vi "GEA3 Determine Valve Absolute Position.vi"(8 "error in (no error)":errorcluster, 9 "Target Position":i16, 11 ".NET Refnum in":refnum<k24>) -> (0 "error out":errorcluster, 1 "Valve Offset":i16, 3 ".NET Refnum out":refnum<k24>, 4 "Previous Mix Valve Position":u16)   [LabVIEW 2016]
uses:
  C:/TechnologyLab/NI-2010/Drivers/GEA3 Toolkit/GEA3 DLL Source/GeaCommunication.dll
  GEA3 DLL Source/GeaCommunication.dll
panel:
  out "Valve Offset Debug":i16
  in  "Current Position Debug":i16
  in  "Target Position Debug":i16
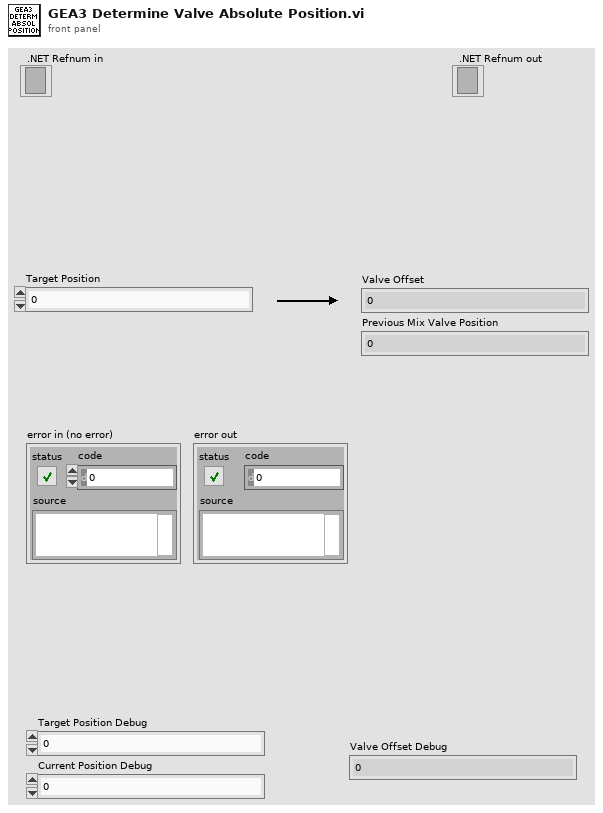
[diagram p1: front panel]
types:
  T1 = typedef "GEA2_Toolkit.lvlib/Source_Destination.ctl" = cluster{"Source":u8, "Destination":u8}
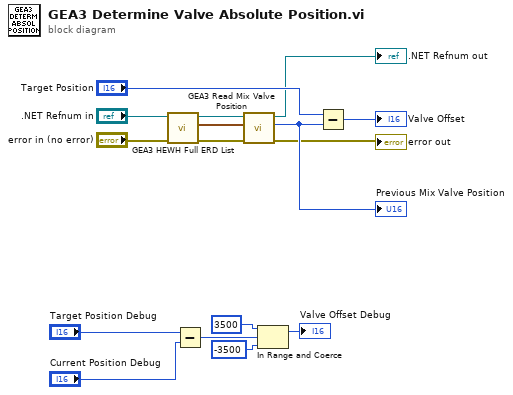
[diagram p0: block diagram]
diagram:
  n1 = call "GEA3 HEWH Full ERD List.vi"("error in (no error)"="error in (no error)", "GEA2 Reference In"=".NET Refnum in") -> ("error out"=w12:errorcluster, "GEA Inputs"=w8:T1, "GEA2 Reference Out"=w11:refnum<k24>)  [unwired: 5 in, 2 out]
  n2 = Subtract(x="Target Position Debug", y="Current Position Debug") -> (x-y=w2:i16)
  n3 = call "GEA3 Read Mix Valve Position.vi"("error in (no error)"=w12, "GEA Inputs"=w8, ".NET Refnum in"=w11) -> ("error out"=→"error out":errorcluster, "Mix Valve Position"=w15:i16, ".NET Refnum out"=→".NET Refnum out":refnum<k24>)  [unwired: 6 in]
  "Previous Mix Valve Position" <- w15
  n4 = In Range and Coerce(upper limit=i16 3500, x=w2, lower limit=i16 -3500) -> (coerced(x)=→"Valve Offset Debug":i16)  [unwired: 1 out]
  n5 = Subtract(x="Target Position", y=w15) -> (x-y=→"Valve Offset":i16)
